vi "EMPEZARGUARDADO.vi"(8 "error in (no error)":errorcluster, 10 "GUARDAR":bool, 11 "GUARDAR_CSV in":refnum<class "GUARDAR_CSV.lvclass">) -> (0 "error out":errorcluster, 3 "GUARDAR_CSV out":refnum<class "GUARDAR_CSV.lvclass">)   [LabVIEW 2019, in "GUARDAR_CSV.lvlib" / "GUARDAR_CSV.lvclass"]
uses:
  GUARDAR_CSV.lvclass
  GUARDAR_CSV.lvclass/GUARDAR_CSV.ctl
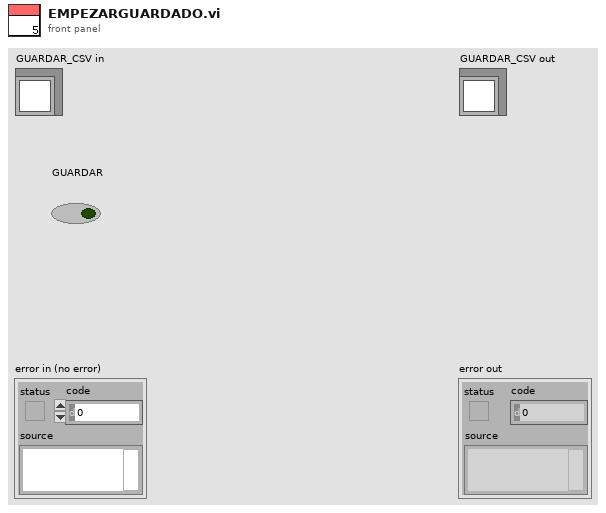
[diagram p1: front panel]
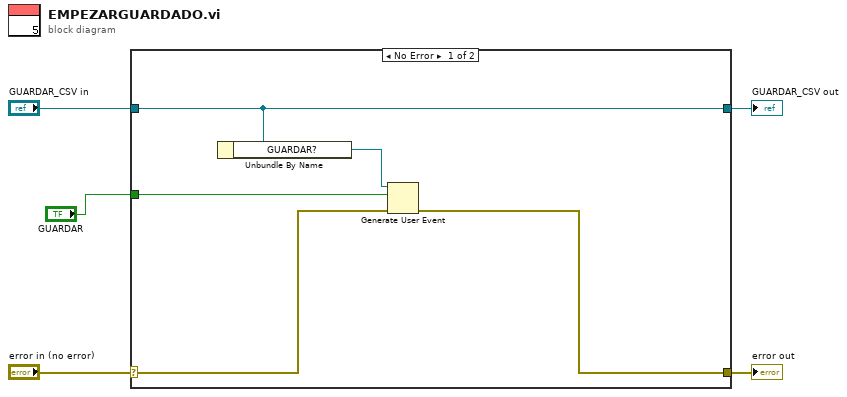
[diagram p0: block diagram]
diagram:
  n1 = case shown="No Error" "error in (no error)" {
    selector: "error in (no error)" -> [w7 w12]
    tunnel: [w6 w12] -> w4
    tunnel: [w10 w11] -> w2
    tunnel: "GUARDAR_CSV in" -> [w10 w11]
    tunnel: "GUARDAR" -> [w8 _]
    frame No Error {
      n2 = Unbundle By Name(w10) -> ("GUARDAR?"=w9:refnum<user-event>)
      n3 = Generate User Event(user event=w9, event data cluster=w8, error in=w7) -> (error out=w6:errorcluster)  [unwired: 1 in, 1 out]
    }
    frame Error {
    }
  }
  "error out" <- w4
  "GUARDAR_CSV out" <- w2
